vi "Write Multiple Holding Registers.vi"(8 "error in (no error)":errorcluster, 9 "holding register values":u16[](array[numeric]), 10 "starting address":u16, 11 "Modbus slave in":refnum<class "Modbus Slave.lvclass">) -> (0 "error out":errorcluster, 3 "Modbus slave out":refnum<class "Modbus Slave.lvclass">)   [LabVIEW 2015, in "Modbus Slave.lvclass"]
doc: "Writes values to contiguous holding registers."
uses:
  <vilib>/Modbus/slave/Modbus Slave.lvclass
  <vilib>/Modbus/slave/Modbus Slave.lvclass/Modbus Slave.ctl
  <vilib>/Modbus/subvis/Data and Functions/Device Data Model/Device Data Model.lvclass
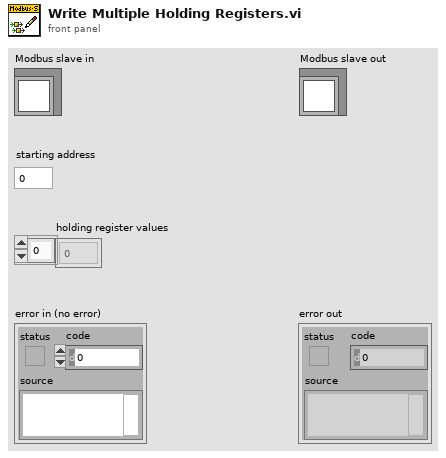
[diagram p1: front panel]
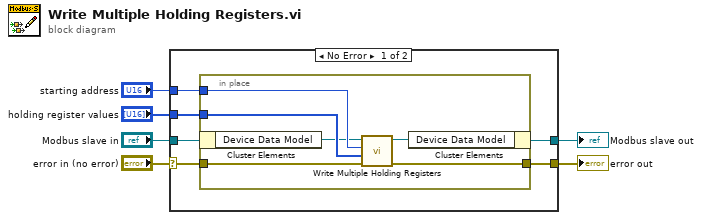
[diagram p0: block diagram]
diagram:
  n1 = case shown="No Error" "error in (no error)" {
    selector: "error in (no error)" -> [w10 w20]
    tunnel: [w9 w20] -> w6
    tunnel: "Modbus slave in" -> [w7 w19]
    tunnel: "holding register values" -> [w12 _]
    tunnel: "starting address" -> [w11 _]
    tunnel: [w8 w19] -> w1
    frame No Error {
      n2 = in-place {
        in-place-border: w12 -> [w18]
        in-place-border: w11 -> [w17]
        in-place-border: w10 -> [w16]
        in-place-border: [w15] -> w9
        n3 = in-place-cluster #1(w7) -> ("Device Data Model"=w14:refnum<class "Device Data Model.lvclass">)
        n4 = call-dynamic "Write Multiple Holding Registers.vi"("error in (no error)"=w16, "register values"=w18, "starting address"=w17, "device data model in"=w14) -> ("error out"=w15:errorcluster, "device data model out"=w13:refnum<class "Device Data Model.lvclass">)  [unwired: 6 in]
        n5 = in-place-cluster #1("Device Data Model"=w13) -> (w8:refnum<class "Modbus Slave.lvclass">)
      }
    }
    frame Error {
    }
  }
  "error out" <- w6
  "Modbus slave out" <- w1
